vi "Register HTTP Handlers.vi"(8 "error in (no error)":errorcluster, 11 "SOL-Server in":refnum<class "SOL-Server.lvclass">) -> (0 "error out":errorcluster, 3 "SOL-Server out":refnum<class "SOL-Server.lvclass">)   [LabVIEW 2020, in "Summer of LabVIEW.lvlib" / "SOL-Server.lvclass"]
uses:
  SOL-Server.lvclass
  Registration/Registration.lvclass
  C:/Program Files (x86)/National Instruments/LabVIEW 2020/vi.lib/IlluminatedG/IG HTTP Server/HTTP Server/Handler/Handler.lvclass
  CSRF/CSRF.lvclass
  User API/User API.lvclass
  Challenges/Challenges.lvclass
  User Submissions API/User Submissions API.lvclass
  Admin Info/Admin Info.lvclass
  SOL-Server.lvclass/SOL-Server.ctl
  Submit/Submit.lvclass
  Error Logger/Error Logger.lvclass
  Approval/Approval.lvclass
  Leaderboard/Leaderboard.lvclass
  <vilib>/IlluminatedG/IG HTTP Server/HTTP Server/Server/Add Connection Handler.vi
  <vilib>/IlluminatedG/IG HTTP Server/HTTP Server/Server/Add Request Handler.vi
  <vilib>/IlluminatedG/IG HTTP Server/HTTP Server/Server/Add Route Handler.vi
  <vilib>/IlluminatedG/IG HTTP Server/HTTP Server/Server/Add Controller Handler.vi
  <vilib>/IlluminatedG/IG HTTP Server/HTTP Server/Server/Add Controller.vi
  <vilib>/IlluminatedG/IG HTTP Server/HTTP Server/Server/Add Response Handler.vi
  <vilib>/IlluminatedG/IG HTTP Server/HTTP Server/Server/Add Complete Handler.vi
  <vilib>/IlluminatedG/IG HTTP Server/HTTP Server/Server/Add Exception Handler.vi
  <vilib>/IlluminatedG/IG HTTP Server/HTTP Server/Connection Handler/Connection Handler.lvclass
  <vilib>/IlluminatedG/IG HTTP Server/HTTP Server/Request Handler/Request Handler.lvclass
  <vilib>/IlluminatedG/IG HTTP Server/HTTP Server/Route Handler/Route Handler.lvclass
  <vilib>/IlluminatedG/IG HTTP Server/HTTP Server/Controller Handler/Controller Handler.lvclass
  <vilib>/IlluminatedG/IG HTTP Server/HTTP Server/Controller/Controller.lvclass
  <vilib>/IlluminatedG/IG HTTP Server/HTTP Server/Response Handler/Response Handler.lvclass
  <vilib>/IlluminatedG/IG HTTP Server/HTTP Server/Complete Handler/Complete Handler.lvclass
  <vilib>/IlluminatedG/IG HTTP Server/HTTP Server/Exception Handler/Exception Handler.lvclass
  <vilib>/IlluminatedG/IG HTTP Server/HTTP Server/Handler/Handler.lvclass
  <vilib>/IlluminatedG/IG HTTP Server/HTTP Server/Server/Server.lvclass
  SOL-Config/SOL-Config.lvclass
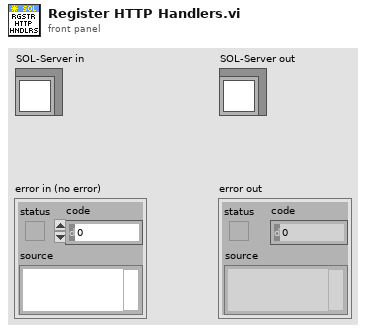
[diagram p1: front panel]
types:
  T1 = typedef "Summer of LabVIEW.lvlib/SOL-Server.lvclass/Paths.ctl" = cluster{"Web Root":path, "Sessions":path, "Config":path, "SQLite DB File":path, "SSL Cert Folder":path, "Submissions":path, "Scorers":path}
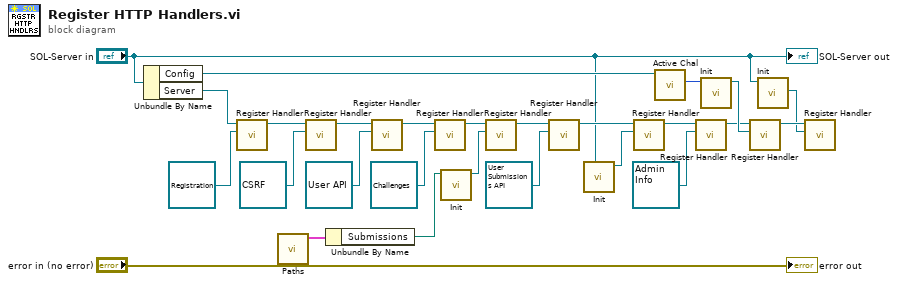
[diagram p0: block diagram]
diagram:
  n1 = Unbundle By Name("SOL-Server in") -> ("Config"=w7:refnum<class "SOL-Config.lvclass">, "Server"=w26:refnum<class "Server.lvclass">)
  n2 = call <vilib>:"Register Handler.vi"("Handler"=refnum<class "Registration.lvclass"> refnum ("SOL:Registration.lvclass"), "Server in"=w26) -> ("Server out"=w23:refnum<class "Server.lvclass">)  [unwired: 8 in, 1 out]
  n3 = call "Paths.vi"() -> ("Paths"=w15:T1)  [unwired: 11 in]
  n4 = call <vilib>:"Register Handler.vi"("Handler"=refnum<class "CSRF.lvclass"> refnum ("SOL:CSRF.lvclass"), "Server in"=w23) -> ("Server out"=w21:refnum<class "Server.lvclass">)  [unwired: 8 in, 1 out]
  n5 = Unbundle By Name(w15) -> ("Submissions"=w14:path)
  n6 = call <vilib>:"Register Handler.vi"("Handler"=refnum<class "User API.lvclass"> refnum ("SOL:User API.lvclass"), "Server in"=w21) -> ("Server out"=w18:refnum<class "Server.lvclass">)  [unwired: 8 in, 1 out]
  n7 = call <vilib>:"Register Handler.vi"("Handler"=refnum<class "Challenges.lvclass"> refnum ("SOL:Challenges.lvclass"), "Server in"=w18) -> ("Server out"=w17:refnum<class "Server.lvclass">)  [unwired: 8 in, 1 out]
  n8 = call "Init.vi"("Submissions"=w14) -> ("Submit out"=w16:refnum<class "Submit.lvclass">)  [unwired: 9 in, 1 out]
  n9 = call <vilib>:"Register Handler.vi"("Handler"=w16, "Server in"=w17) -> ("Server out"=w13:refnum<class "Server.lvclass">)  [unwired: 8 in, 1 out]
  n10 = call <vilib>:"Register Handler.vi"("Handler"=refnum<class "User Submissions API.lvclass"> refnum ("SOL:User Submissions API.lvclass"), "Server in"=w13) -> ("Server out"=w11:refnum<class "Server.lvclass">)  [unwired: 8 in, 1 out]
  n11 = call "Init.vi"("SoL Server"="SOL-Server in") -> ("Approval out"=w8:refnum<class "Approval.lvclass">)  [unwired: 9 in, 1 out]
  n12 = call <vilib>:"Register Handler.vi"("Handler"=w8, "Server in"=w11) -> ("Server out"=w10:refnum<class "Server.lvclass">)  [unwired: 8 in, 1 out]
  n13 = call "Active Chal.vi"("SOL-Config in"=w7) -> ("Active Chal"=w6:i64)  [unwired: 8 in, 2 out]
  n14 = call <vilib>:"Register Handler.vi"("Handler"=refnum<class "Admin Info.lvclass"> refnum ("SOL:Pending Submissions.lvclass"), "Server in"=w10) -> ("Server out"=w4:refnum<class "Server.lvclass">)  [unwired: 8 in, 1 out]
  n15 = call "Init.vi"("Active Chal ID"=w6) -> ("Scores out"=w5:refnum<class "Leaderboard.lvclass">)  [unwired: 9 in, 1 out]
  n16 = call <vilib>:"Register Handler.vi"("Handler"=w5, "Server in"=w4) -> ("Server out"=w3:refnum<class "Server.lvclass">)  [unwired: 8 in, 1 out]
  n17 = call "Init.vi"("SOL Server"="SOL-Server in") -> ("Error Logger out"=w2:refnum<class "Error Logger.lvclass">)  [unwired: 9 in, 1 out]
  n18 = call <vilib>:"Register Handler.vi"("Handler"=w2, "Server in"=w3) -> ()  [unwired: 8 in, 2 out]
  "error out" <- "error in (no error)"
  "SOL-Server out" <- "SOL-Server in"
